vi "WFAppend2D.vi"(4 "error in (no error)":errorcluster, 6 "Waveform In 2":digitalwaveform(waveform)={"t0"=timestamp(0 s since 1904-01-01), "dt"=1.0, "Y"={"transitions"=[], "data"=[]}}, 7 "Waveform In":digitalwaveform(waveform)={"t0"=timestamp(0 s since 1904-01-01), "dt"=1.0, "Y"={"transitions"=[], "data"=[]}}) -> (0 "error out":errorcluster, 3 "Waveform Out":digitalwaveform(waveform)={"t0"=timestamp(0 s since 1904-01-01), "dt"=1.0, "Y"={"transitions"=[], "data"=[]}})   [LabVIEW 2013]
uses:
  <vilib>/Waveform/DWDTOps.llb/DWDT Digital Size.vi
  <vilib>/Waveform/DWDTOps.llb/DWDT Append Digital Samples.vi
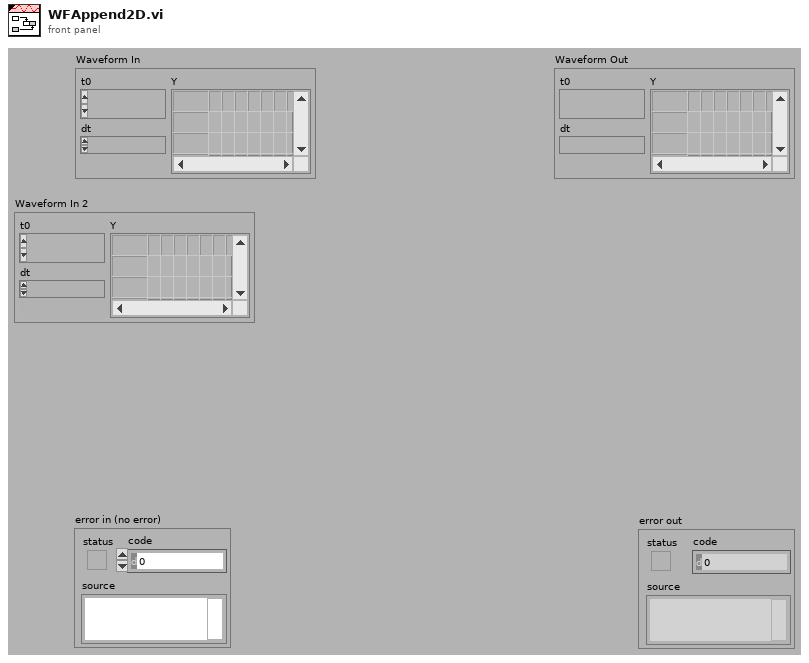
[diagram p1: front panel]
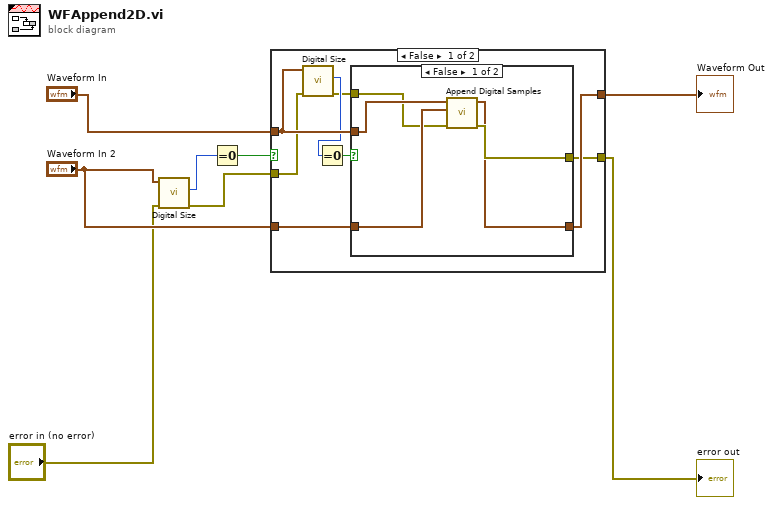
[diagram p0: block diagram]
diagram:
  n1 = call-poly <vilib>:"Digital Size.vi"("error in (no error)"="error in (no error)", "digital waveform in"="Waveform In 2") -> ("error out"=w1:errorcluster, "number of samples"=w2:i32)  [unwired: 6 in, 2 out]
  n2 = Equal To 0?(x=w2) -> (x = 0?=w8:bool)
  n3 = case shown="False" w8 {
    tunnel: "Waveform In" -> [w12 w25]
    tunnel: "Waveform In 2" -> [w15 _]
    tunnel: [w14 w25] -> w6
    tunnel: w1 -> [w11 w24]
    tunnel: [w13 w24] -> w5
    frame False {
      n4 = call-poly <vilib>:"Digital Size.vi"("error in (no error)"=w11, "digital waveform in"=w12) -> ("error out"=w9:errorcluster, "number of samples"=w10:i32)  [unwired: 6 in, 2 out]
      n5 = Equal To 0?(x=w10) -> (x = 0?=w16:bool)
      n6 = case shown="False" w16 {
        tunnel: [w17 w23] -> w14
        tunnel: w15 -> [w20 w23]
        tunnel: w12 -> [w21 _]
        tunnel: [w18 w22] -> w13
        tunnel: w9 -> [w19 w22]
        frame False {
          n7 = call-poly <vilib>:"Append Digital Samples.vi"("error in (no error)"=w19, "digital waveform B"=w20, "digital waveform A"=w21) -> ("error out"=w18:errorcluster, "digital waveform out"=w17:digitalwaveform)  [unwired: 7 in]
        }
        frame True {
        }
      }
    }
    frame True {
    }
  }
  "Waveform Out" <- w6
  "error out" <- w5
